vi "PixelDetection.vi"(9 "Key input":T1, 10 "Level input":u32[][](array[colorbox]), 11 "Location input":cluster{"Y":i32, "X":i32}[](array[cluster])=[{"Y"=10, "X"=5}]) -> (1 "Key output":T1, 2 "Level output":u32[][](array[colorbox]), 3 "Location output":cluster{"Y":i32, "X":i32}[](array[cluster])=[{"Y"=10, "X"=5}], 4 "Food eaten?":bool, 5 "Game Over?":bool)   [LabVIEW 2021]
uses:
  TypeDef/KeyDown.ctl
  GlobalVariables/Board_Colors.vi
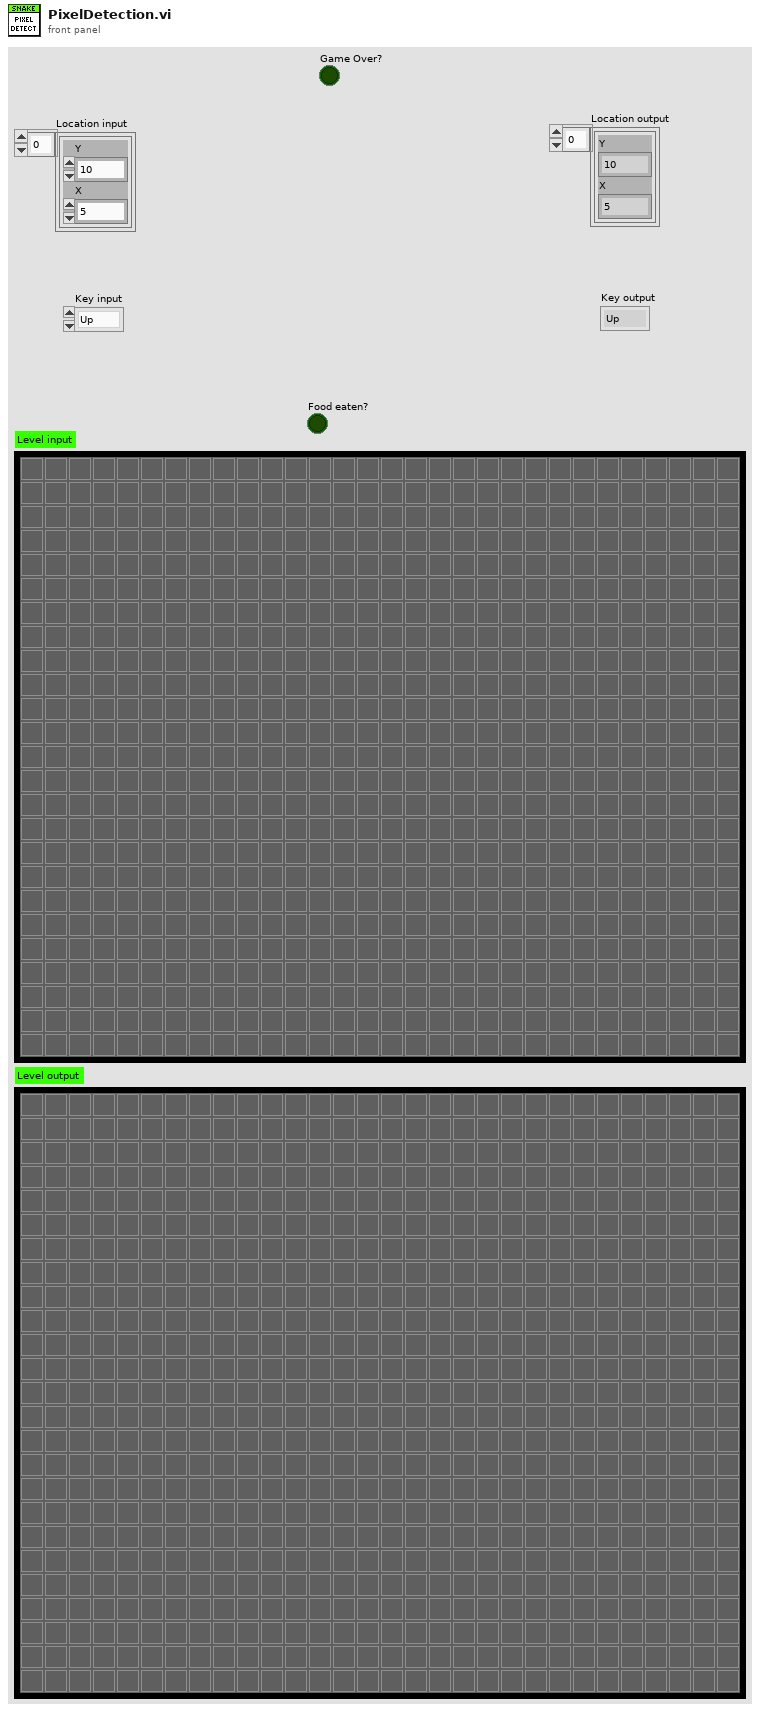
[diagram p1: front panel]
types:
  T1 = typedef "KeyDown.ctl" = enum16{"Up", "Down", "Left", "Right"}
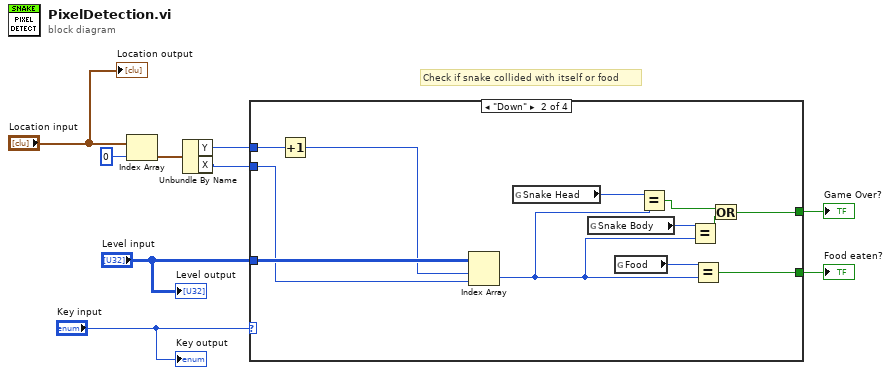
[diagram p0: block diagram]
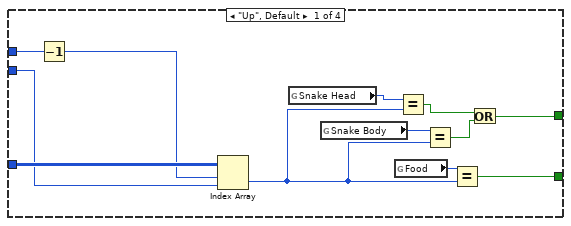
[diagram p2: hidden frame]
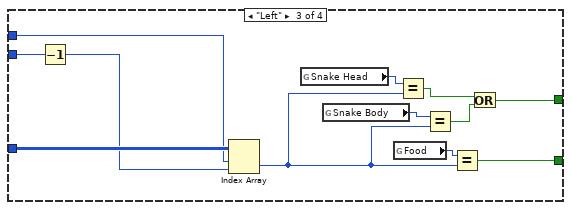
[diagram p3: hidden frame]
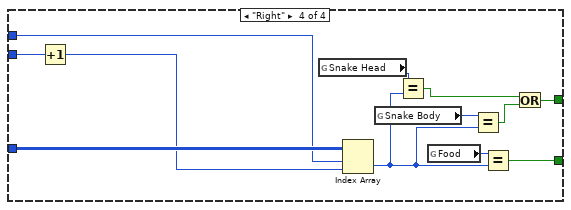
[diagram p4: hidden frame]
diagram:
  # "Check if snake collided with itself or food"
  n1 = Index Array(array="Location input", index=0) -> (element=w6:cluster{"Y":i32, "X":i32})
  n2 = Unbundle By Name(w6) -> ("Y"=w5:i32, "X"=w4:i32)
  n3 = case shown="\"Down\"" "Key input" {
    tunnel: w5 -> [w21 w33 w39 w51]
    tunnel: w4 -> [w19 w31 w38 w50]
    tunnel: "Level input" -> [w20 w32 w45 w57]
    tunnel: [w17 w29 w43 w55] -> w2
    tunnel: [w14 w26 w40 w52] -> w1
    frame "Up", Default {
      n4 = Decrement(x=w21) -> (x-1=w13:i32)
      n5 = Index Array(array=w20, index (row)=w13, index (col)=w19) -> (element=w18:u32)
      n6 = global read "Board_Colors.vi" "Snake Head"() -> (w10:u32)
      n7 = global read "Board_Colors.vi" "Snake Body"() -> (w11:u32)
      n8 = global read "Board_Colors.vi" "Food"() -> (w12:u32)
      n9 = Equal?(x=w10, y=w18) -> (x = y?=w15:bool)
      n10 = Equal?(x=w11, y=w18) -> (x = y?=w16:bool)
      n11 = Equal?(x=w12, y=w18) -> (x = y?=w17:bool)
      n12 = Or(x=w15, y=w16) -> (x .or. y?=w14:bool)
    }
    frame "Down" {
      n13 = Increment(x=w33) -> (x+1=w25:i32)
      n14 = Index Array(array=w32, index (row)=w25, index (col)=w31) -> (element=w30:u32)
      n15 = global read "Board_Colors.vi" "Snake Head"() -> (w24:u32)
      n16 = global read "Board_Colors.vi" "Snake Body"() -> (w23:u32)
      n17 = global read "Board_Colors.vi" "Food"() -> (w22:u32)
      n18 = Equal?(x=w24, y=w30) -> (x = y?=w27:bool)
      n19 = Equal?(x=w23, y=w30) -> (x = y?=w28:bool)
      n20 = Equal?(x=w22, y=w30) -> (x = y?=w29:bool)
      n21 = Or(x=w27, y=w28) -> (x .or. y?=w26:bool)
    }
    frame "Left" {
      n22 = Decrement(x=w38) -> (x-1=w37:i32)
      n23 = Index Array(array=w45, index (row)=w39, index (col)=w37) -> (element=w44:u32)
      n24 = global read "Board_Colors.vi" "Snake Head"() -> (w34:u32)
      n25 = global read "Board_Colors.vi" "Snake Body"() -> (w35:u32)
      n26 = global read "Board_Colors.vi" "Food"() -> (w36:u32)
      n27 = Equal?(x=w34, y=w44) -> (x = y?=w41:bool)
      n28 = Equal?(x=w35, y=w44) -> (x = y?=w42:bool)
      n29 = Equal?(x=w36, y=w44) -> (x = y?=w43:bool)
      n30 = Or(x=w41, y=w42) -> (x .or. y?=w40:bool)
    }
    frame "Right" {
      n31 = Increment(x=w50) -> (x+1=w46:i32)
      n32 = global read "Board_Colors.vi" "Snake Head"() -> (w48:u32)
      n33 = Index Array(array=w57, index (row)=w51, index (col)=w46) -> (element=w56:u32)
      n34 = global read "Board_Colors.vi" "Snake Body"() -> (w47:u32)
      n35 = Equal?(x=w48, y=w56) -> (x = y?=w53:bool)
      n36 = global read "Board_Colors.vi" "Food"() -> (w49:u32)
      n37 = Equal?(x=w47, y=w56) -> (x = y?=w54:bool)
      n38 = Equal?(x=w49, y=w56) -> (x = y?=w55:bool)
      n39 = Or(x=w53, y=w54) -> (x .or. y?=w52:bool)
    }
  }
  "Food eaten?" <- w2
  "Game Over?" <- w1
  "Key output" <- "Key input"
  "Location output" <- "Location input"
  "Level output" <- "Level input"
